vi "Send_Window.vi"(10 "Iteration":i32, 11 "Data Sample":dbl[](array[numeric])) -> (3 "Boolean":bool)   [LabVIEW 2020]
uses:
  Global Variables/Window_Size.vi
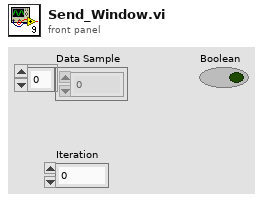
[diagram p1: front panel]
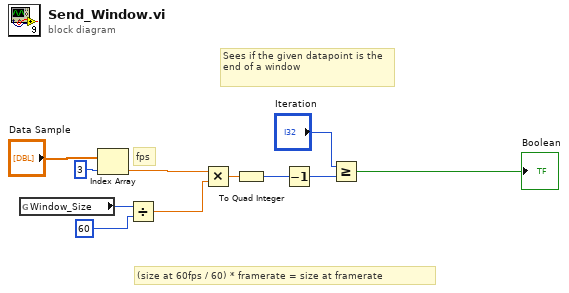
[diagram p0: block diagram]
diagram:
  # "(size at 60fps / 60) * framerate = size at framerate"
  # "fps"
  # "Sees if the given datapoint is the end of a window"
  n1 = global read "Window_Size.vi" "Window_Size"() -> (w3:i64)
  n2 = Index Array(array="Data Sample", index=3) -> (element=w7:dbl)
  n3 = Divide(x=w3, y=60) -> (x/y=w1:dbl)
  n4 = Multiply(x=w7, y=w1) -> (x*y=w5:dbl)
  n5 = To Quad Integer(1:w5) -> (0:w8:i64)
  n6 = Decrement(x=w8) -> (x-1=w9:i64)
  n7 = Greater Or Equal?(x="Iteration", y=w9) -> (x >= y?=→"Boolean":bool)
